vi "CoOpStackOnTwo.vi"(11 "Array":bool[](array[boolean])) -> ()   [LabVIEW 2014]
uses:
  CoOpStackOnTwo.ctl
  Gantry/GantryGlobals.vi
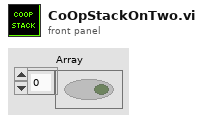
[diagram p1: front panel]
types:
  T1 = typedef "CoOpStackOnTwo.ctl" = enum16{"WaitingForInput", "OpenArms", "PlaceOnNone", "CloseArms", "Lift", "GantryOut", "LowerArms", "OpenArms2", "GantryIn"}
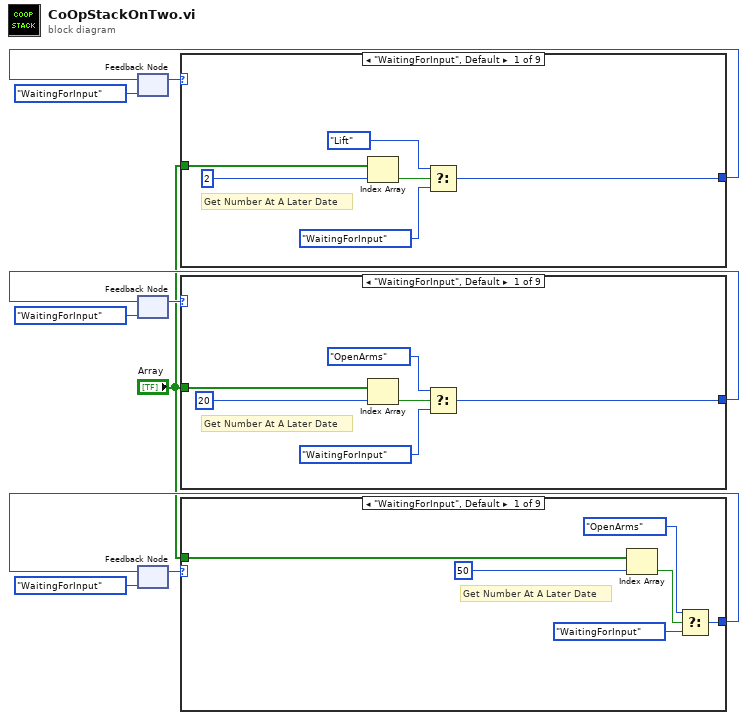
[diagram p0: block diagram]
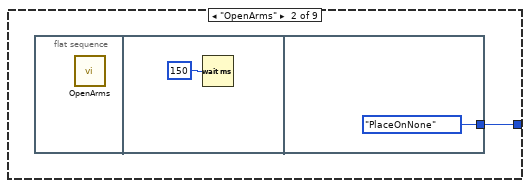
[diagram p2: hidden frame]
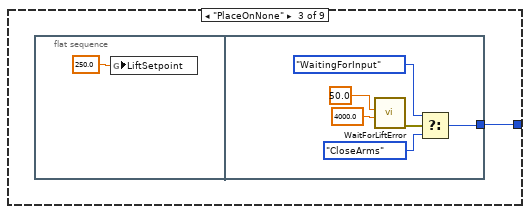
[diagram p3: hidden frame]
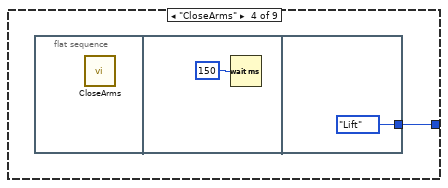
[diagram p4: hidden frame]
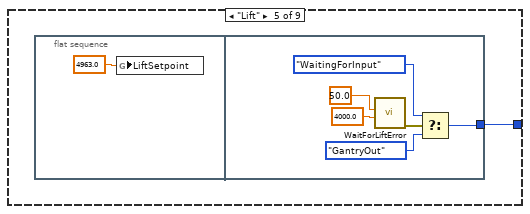
[diagram p5: hidden frame]
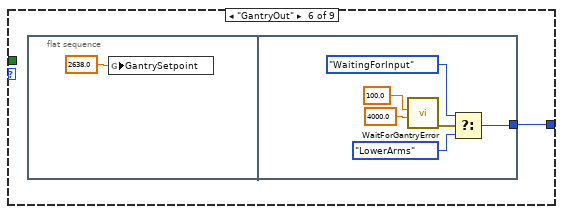
[diagram p6: hidden frame]
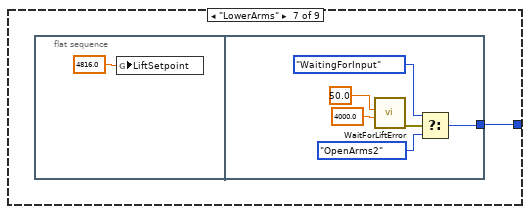
[diagram p7: hidden frame]
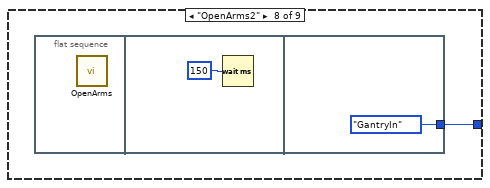
[diagram p8: hidden frame]
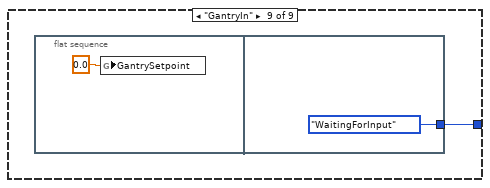
[diagram p9: hidden frame]
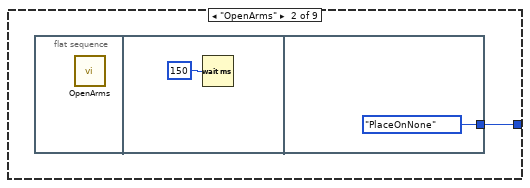
[diagram p10: hidden frame]
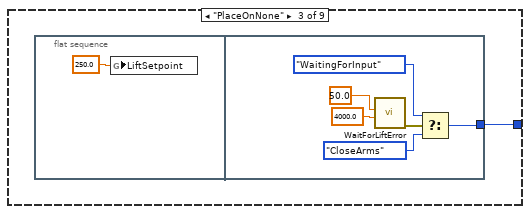
[diagram p11: hidden frame]
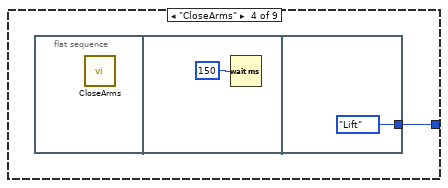
[diagram p12: hidden frame]
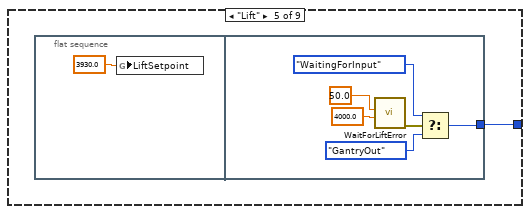
[diagram p13: hidden frame]
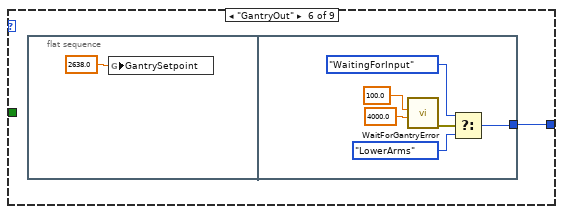
[diagram p14: hidden frame]
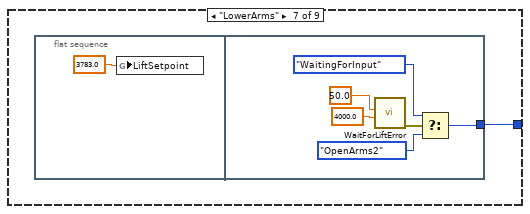
[diagram p15: hidden frame]
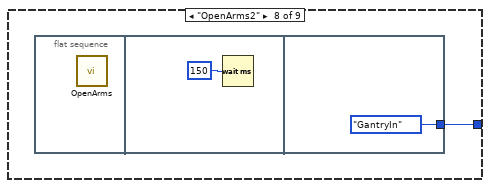
[diagram p16: hidden frame]
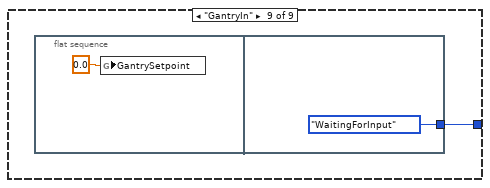
[diagram p17: hidden frame]
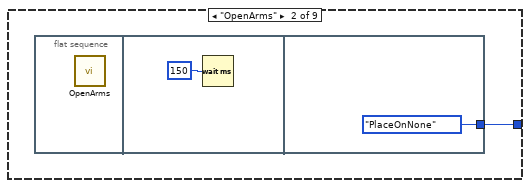
[diagram p18: hidden frame]
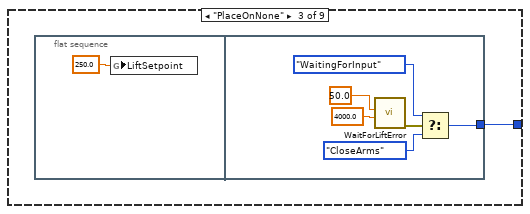
[diagram p19: hidden frame]
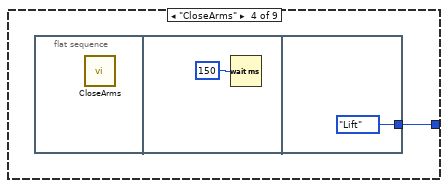
[diagram p20: hidden frame]
diagram:
  n1 = feedback #1(CoOpStackOnTwo."WaitingForInput" ("CoOpStackOn2")) -> (w10:T1)
  n2 = feedback #2(CoOpStackOnTwo."WaitingForInput" ("CoOpStackOn2")) -> (w7:T1)
  n3 = feedback #3(CoOpStackOnTwo."WaitingForInput" ("CoOpStackOn2")) -> (w2:T1)
  n4 = case shown="\"WaitingForInput\", Default" w10 {
    tunnel: "Array" -> [w15 _ _ _ _ _ _ _ _]
    tunnel: [w11 w17 w20 w28 w31 w39 w47 w55 w58] -> w8
    frame "WaitingForInput", Default {
      # "Get Number At A Later Date"
      n5 = Index Array(array=w15, index=2) -> (element=w14:bool)
      n6 = Select(t=CoOpStackOnTwo."Lift" ("CoOpStackOn2"), s=w14, f=CoOpStackOnTwo."WaitingForInput" ("CoOpStackOn2")) -> (s? t:f=w11:T1)
    }
    frame "OpenArms" {
      n7 = flat-sequence {
        tunnel: [CoOpStackOnTwo."PlaceOnNone" ("CoOpStackOn2")] -> w17
        frame #0 {
          n8 = call "OpenArms.vi"() -> ()  [unwired: 12 in]
        }
        frame #1 {
          n9 = Wait (ms)(milliseconds to wait=u32 150) -> ()  [unwired: 1 out]
        }
        frame #2 {
        }
      }
    }
    frame "PlaceOnNone" {
      n10 = flat-sequence {
        tunnel: [w22] -> w20
        frame #0 {
          n11 = global write "GantryGlobals.vi" "LiftSetpoint"(250.0 ("LiftSetpoint")) -> ()
        }
        frame #1 {
          n12 = call "WaitForLiftError.vi"("Timeout (ms)"=4000.0, "AllowedError"=50.0) -> ("error out"=w25:errorcluster)  [unwired: 9 in]
          n13 = Select(t=CoOpStackOnTwo."WaitingForInput" ("CoOpStackOn2"), s=w25, f=CoOpStackOnTwo."CloseArms" ("CoOpStackOn2")) -> (s? t:f=w22:T1)
        }
      }
    }
    frame "CloseArms" {
      n14 = flat-sequence {
        tunnel: [CoOpStackOnTwo."Lift" ("CoOpStackOn2")] -> w28
        frame #0 {
          n15 = call "CloseArms.vi"() -> ()  [unwired: 12 in]
        }
        frame #1 {
          n16 = Wait (ms)(milliseconds to wait=u32 150) -> ()  [unwired: 1 out]
        }
        frame #2 {
        }
      }
    }
    frame "Lift" {
      n17 = flat-sequence {
        tunnel: [w33] -> w31
        frame #0 {
          # "Value is TBD"
          n18 = global write "GantryGlobals.vi" "LiftSetpoint"(270.0 ("LiftSetpoint")) -> ()
        }
        frame #1 {
          n19 = call "WaitForLiftError.vi"("Timeout (ms)"=3000.0, "AllowedError"=3.0) -> ("error out"=w36:errorcluster)  [unwired: 9 in]
          n20 = Select(t=CoOpStackOnTwo."WaitingForInput" ("CoOpStackOn2"), s=w36, f=CoOpStackOnTwo."GantryOut" ("CoOpStackOn2")) -> (s? t:f=w33:T1)
        }
      }
    }
    frame "GantryOut" {
      n21 = flat-sequence {
        tunnel: [w41] -> w39
        frame #0 {
          n22 = global write "GantryGlobals.vi" "GantrySetpoint"(2638.0 ("GantrySetpoint")) -> ()
        }
        frame #1 {
          n23 = call "WaitForGantryError.vi"("Timeout (ms)"=4000.0, "AllowedError"=100.0) -> ("error out"=w44:errorcluster)  [unwired: 9 in]
          n24 = Select(t=CoOpStackOnTwo."WaitingForInput" ("CoOpStackOn2"), s=w44, f=CoOpStackOnTwo."LowerArms" ("CoOpStackOn2")) -> (s? t:f=w41:T1)
        }
      }
    }
    frame "LowerArms" {
      n25 = flat-sequence {
        tunnel: [w49] -> w47
        frame #0 {
          n26 = global write "GantryGlobals.vi" "LiftSetpoint"(260.0 ("LiftSetpoint")) -> ()
        }
        frame #1 {
          n27 = call "WaitForLiftError.vi"("Timeout (ms)"=3000.0, "AllowedError"=3.0) -> ("error out"=w52:errorcluster)  [unwired: 9 in]
          n28 = Select(t=CoOpStackOnTwo."WaitingForInput" ("CoOpStackOn2"), s=w52, f=CoOpStackOnTwo."OpenArms2" ("CoOpStackOn2")) -> (s? t:f=w49:T1)
        }
      }
    }
    frame "OpenArms2" {
      n29 = flat-sequence {
        tunnel: [CoOpStackOnTwo."GantryIn" ("CoOpStackOn2")] -> w55
        frame #0 {
          n30 = call "OpenArms.vi"() -> ()  [unwired: 12 in]
        }
        frame #1 {
          n31 = Wait (ms)(milliseconds to wait=u32 150) -> ()  [unwired: 1 out]
        }
        frame #2 {
        }
      }
    }
    frame "GantryIn" {
      n32 = flat-sequence {
        tunnel: [CoOpStackOnTwo."WaitingForInput" ("CoOpStackOn2")] -> w58
        frame #0 {
          n33 = global write "GantryGlobals.vi" "GantrySetpoint"(0.0 ("GantrySetpoint")) -> ()
        }
        frame #1 {
        }
      }
    }
  }
  n34 = feedback-in #1(w8) -> ()
  n35 = case shown="\"WaitingForInput\", Default" w7 {
    tunnel: "Array" -> [w65 _ _ _ _ _ _ _ _]
    tunnel: [w61 w67 w70 w78 w81 w89 w97 w105 w108] -> w5
    frame "WaitingForInput", Default {
      # "Get Number At A Later Date"
      n36 = Index Array(array=w65, index=20) -> (element=w64:bool)
      n37 = Select(t=CoOpStackOnTwo."OpenArms" ("CoOpStackOn2"), s=w64, f=CoOpStackOnTwo."WaitingForInput" ("CoOpStackOn2")) -> (s? t:f=w61:T1)
    }
    frame "OpenArms" {
      n38 = flat-sequence {
        tunnel: [CoOpStackOnTwo."PlaceOnNone" ("CoOpStackOn2")] -> w67
        frame #0 {
          n39 = call "OpenArms.vi"() -> ()  [unwired: 12 in]
        }
        frame #1 {
          n40 = Wait (ms)(milliseconds to wait=u32 150) -> ()  [unwired: 1 out]
        }
        frame #2 {
        }
      }
    }
    frame "PlaceOnNone" {
      n41 = flat-sequence {
        tunnel: [w72] -> w70
        frame #0 {
          n42 = global write "GantryGlobals.vi" "LiftSetpoint"(250.0 ("LiftSetpoint")) -> ()
        }
        frame #1 {
          n43 = call "WaitForLiftError.vi"("Timeout (ms)"=4000.0, "AllowedError"=50.0) -> ("error out"=w75:errorcluster)  [unwired: 9 in]
          n44 = Select(t=CoOpStackOnTwo."WaitingForInput" ("CoOpStackOn2"), s=w75, f=CoOpStackOnTwo."CloseArms" ("CoOpStackOn2")) -> (s? t:f=w72:T1)
        }
      }
    }
    frame "CloseArms" {
      n45 = flat-sequence {
        tunnel: [CoOpStackOnTwo."Lift" ("CoOpStackOn2")] -> w78
        frame #0 {
          n46 = call "CloseArms.vi"() -> ()  [unwired: 12 in]
        }
        frame #1 {
          n47 = Wait (ms)(milliseconds to wait=u32 150) -> ()  [unwired: 1 out]
        }
        frame #2 {
        }
      }
    }
    frame "Lift" {
      n48 = flat-sequence {
        tunnel: [w83] -> w81
        frame #0 {
          n49 = global write "GantryGlobals.vi" "LiftSetpoint"(3930.0 ("LiftSetpoint")) -> ()
        }
        frame #1 {
          n50 = call "WaitForLiftError.vi"("Timeout (ms)"=4000.0, "AllowedError"=50.0) -> ("error out"=w86:errorcluster)  [unwired: 9 in]
          n51 = Select(t=CoOpStackOnTwo."WaitingForInput" ("CoOpStackOn2"), s=w86, f=CoOpStackOnTwo."GantryOut" ("CoOpStackOn2")) -> (s? t:f=w83:T1)
        }
      }
    }
    frame "GantryOut" {
      n52 = flat-sequence {
        tunnel: [w91] -> w89
        frame #0 {
          n53 = global write "GantryGlobals.vi" "GantrySetpoint"(2638.0 ("GantrySetpoint")) -> ()
        }
        frame #1 {
          n54 = call "WaitForGantryError.vi"("Timeout (ms)"=4000.0, "AllowedError"=100.0) -> ("error out"=w94:errorcluster)  [unwired: 9 in]
          n55 = Select(t=CoOpStackOnTwo."WaitingForInput" ("CoOpStackOn2"), s=w94, f=CoOpStackOnTwo."LowerArms" ("CoOpStackOn2")) -> (s? t:f=w91:T1)
        }
      }
    }
    frame "LowerArms" {
      n56 = flat-sequence {
        tunnel: [w99] -> w97
        frame #0 {
          n57 = global write "GantryGlobals.vi" "LiftSetpoint"(3783.0 ("LiftSetpoint")) -> ()
        }
        frame #1 {
          n58 = call "WaitForLiftError.vi"("Timeout (ms)"=4000.0, "AllowedError"=50.0) -> ("error out"=w102:errorcluster)  [unwired: 9 in]
          n59 = Select(t=CoOpStackOnTwo."WaitingForInput" ("CoOpStackOn2"), s=w102, f=CoOpStackOnTwo."OpenArms2" ("CoOpStackOn2")) -> (s? t:f=w99:T1)
        }
      }
    }
    frame "OpenArms2" {
      n60 = flat-sequence {
        tunnel: [CoOpStackOnTwo."GantryIn" ("CoOpStackOn2")] -> w105
        frame #0 {
          n61 = call "OpenArms.vi"() -> ()  [unwired: 12 in]
        }
        frame #1 {
          n62 = Wait (ms)(milliseconds to wait=u32 150) -> ()  [unwired: 1 out]
        }
        frame #2 {
        }
      }
    }
    frame "GantryIn" {
      n63 = flat-sequence {
        tunnel: [CoOpStackOnTwo."WaitingForInput" ("CoOpStackOn2")] -> w108
        frame #0 {
          n64 = global write "GantryGlobals.vi" "GantrySetpoint"(0.0 ("GantrySetpoint")) -> ()
        }
        frame #1 {
        }
      }
    }
  }
  n65 = feedback-in #2(w5) -> ()
  n66 = case shown="\"WaitingForInput\", Default" w2 {
    tunnel: [w113 w117 w120 w128 w131 w139 w147 w155 w158] -> w4
    tunnel: "Array" -> [w112 _ _ _ _ _ _ _ _]
    frame "WaitingForInput", Default {
      # "Get Number At A Later Date"
      n67 = Index Array(array=w112, index=50) -> (element=w111:bool)
      n68 = Select(t=CoOpStackOnTwo."OpenArms" ("CoOpStackOn2"), s=w111, f=CoOpStackOnTwo."WaitingForInput" ("CoOpStackOn2")) -> (s? t:f=w113:T1)
    }
    frame "OpenArms" {
      n69 = flat-sequence {
        tunnel: [CoOpStackOnTwo."PlaceOnNone" ("CoOpStackOn2")] -> w117
        frame #0 {
          n70 = call "OpenArms.vi"() -> ()  [unwired: 12 in]
        }
        frame #1 {
          n71 = Wait (ms)(milliseconds to wait=u32 150) -> ()  [unwired: 1 out]
        }
        frame #2 {
        }
      }
    }
    frame "PlaceOnNone" {
      n72 = flat-sequence {
        tunnel: [w122] -> w120
        frame #0 {
          n73 = global write "GantryGlobals.vi" "LiftSetpoint"(250.0 ("LiftSetpoint")) -> ()
        }
        frame #1 {
          n74 = call "WaitForLiftError.vi"("Timeout (ms)"=4000.0, "AllowedError"=50.0) -> ("error out"=w125:errorcluster)  [unwired: 9 in]
          n75 = Select(t=CoOpStackOnTwo."WaitingForInput" ("CoOpStackOn2"), s=w125, f=CoOpStackOnTwo."CloseArms" ("CoOpStackOn2")) -> (s? t:f=w122:T1)
        }
      }
    }
    frame "CloseArms" {
      n76 = flat-sequence {
        tunnel: [CoOpStackOnTwo."Lift" ("CoOpStackOn2")] -> w128
        frame #0 {
          n77 = call "CloseArms.vi"() -> ()  [unwired: 12 in]
        }
        frame #1 {
          n78 = Wait (ms)(milliseconds to wait=u32 150) -> ()  [unwired: 1 out]
        }
        frame #2 {
        }
      }
    }
    frame "Lift" {
      n79 = flat-sequence {
        tunnel: [w133] -> w131
        frame #0 {
          n80 = global write "GantryGlobals.vi" "LiftSetpoint"(4963.0 ("LiftSetpoint")) -> ()
        }
        frame #1 {
          n81 = call "WaitForLiftError.vi"("Timeout (ms)"=4000.0, "AllowedError"=50.0) -> ("error out"=w136:errorcluster)  [unwired: 9 in]
          n82 = Select(t=CoOpStackOnTwo."WaitingForInput" ("CoOpStackOn2"), s=w136, f=CoOpStackOnTwo."GantryOut" ("CoOpStackOn2")) -> (s? t:f=w133:T1)
        }
      }
    }
    frame "GantryOut" {
      n83 = flat-sequence {
        tunnel: [w141] -> w139
        frame #0 {
          n84 = global write "GantryGlobals.vi" "GantrySetpoint"(2638.0 ("GantrySetpoint")) -> ()
        }
        frame #1 {
          n85 = call "WaitForGantryError.vi"("Timeout (ms)"=4000.0, "AllowedError"=100.0) -> ("error out"=w144:errorcluster)  [unwired: 9 in]
          n86 = Select(t=CoOpStackOnTwo."WaitingForInput" ("CoOpStackOn2"), s=w144, f=CoOpStackOnTwo."LowerArms" ("CoOpStackOn2")) -> (s? t:f=w141:T1)
        }
      }
    }
    frame "LowerArms" {
      n87 = flat-sequence {
        tunnel: [w149] -> w147
        frame #0 {
          n88 = global write "GantryGlobals.vi" "LiftSetpoint"(4816.0 ("LiftSetpoint")) -> ()
        }
        frame #1 {
          n89 = call "WaitForLiftError.vi"("Timeout (ms)"=4000.0, "AllowedError"=50.0) -> ("error out"=w152:errorcluster)  [unwired: 9 in]
          n90 = Select(t=CoOpStackOnTwo."WaitingForInput" ("CoOpStackOn2"), s=w152, f=CoOpStackOnTwo."OpenArms2" ("CoOpStackOn2")) -> (s? t:f=w149:T1)
        }
      }
    }
    frame "OpenArms2" {
      n91 = flat-sequence {
        tunnel: [CoOpStackOnTwo."GantryIn" ("CoOpStackOn2")] -> w155
        frame #0 {
          n92 = call "OpenArms.vi"() -> ()  [unwired: 12 in]
        }
        frame #1 {
          n93 = Wait (ms)(milliseconds to wait=u32 150) -> ()  [unwired: 1 out]
        }
        frame #2 {
        }
      }
    }
    frame "GantryIn" {
      n94 = flat-sequence {
        tunnel: [CoOpStackOnTwo."WaitingForInput" ("CoOpStackOn2")] -> w158
        frame #0 {
          n95 = global write "GantryGlobals.vi" "GantrySetpoint"(0.0 ("GantrySetpoint")) -> ()
        }
        frame #1 {
        }
      }
    }
  }
  n96 = feedback-in #3(w4) -> ()
